vi "Update Params.vi"(6 "EccFileName":string="ocv4.ecc", 7 "Params":T1(array[cluster]), 8 "error in (no error)":errorcluster, 9 "TechIndex":i32, 10 "Channel":u8, 11 "ID":i32) -> (0 "error out":errorcluster, 3 "ID Out":i32)   [LabVIEW 2022 SP3, in "EClib functions.lvlib"]
doc: "This VI stops loaded ecc protocols on the selected channel."
uses:
  EClib functions.lvlib
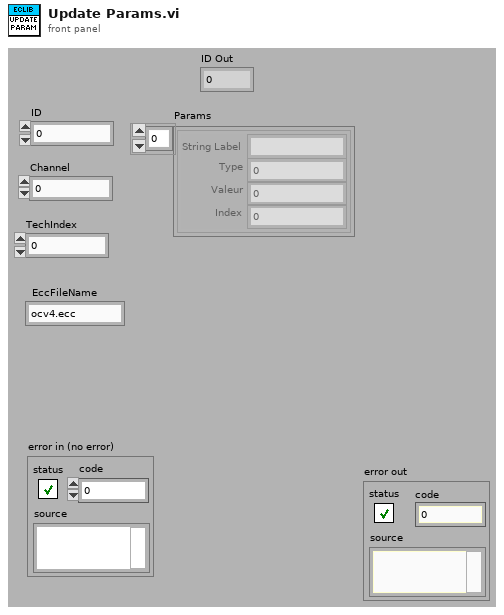
[diagram p1: front panel]
types:
  T1 = cluster{"String Label":string, "Type":i32, "Valeur":i32, "Index":i32}[]
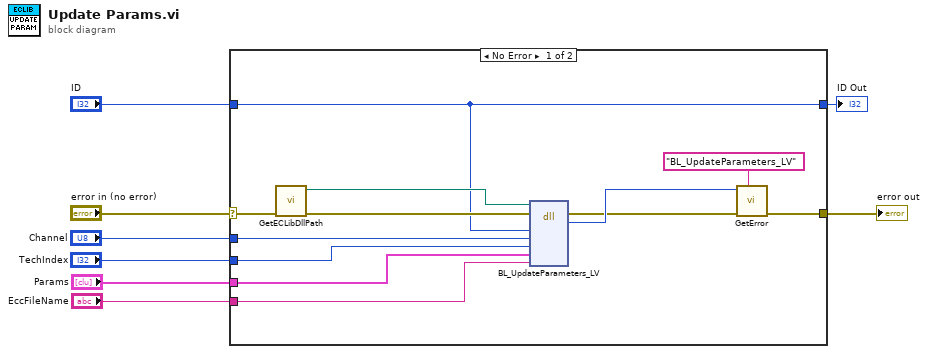
[diagram p0: block diagram]
diagram:
  n1 = case shown="No Error" "error in (no error)" {
    selector: "error in (no error)" -> [w14 w22]
    tunnel: [w19 w22] -> w8
    tunnel: "Params" -> [w13 _]
    tunnel: "TechIndex" -> [w12 _]
    tunnel: "Channel" -> [w11 _]
    tunnel: "EccFileName" -> [w10 _]
    tunnel: "ID" -> [w9 w21]
    tunnel: [w9 w21] -> w1
    frame No Error {
      n2 = call "GetECLibDllPath.vi"("error in (no error)"=w14) -> ("error out"=w15:errorcluster, "ECLibDLLPath"=w20:path)  [unwired: 9 in]
      n3 = dll-call lib="?" fn="BL_UpdateParameters_LV"(path in=w20, error in=w15, "ID"=w9, "Channel"=w11, "TechIndex"=w12, "Params"=w13, "EccFileName"=w10) -> (error out=w16:errorcluster, "return type"=w18:i32)  [unwired: 6 in, 1 out]
      n4 = call "GetError.vi"("DLLFunction"="BL_UpdateParameters_LV", "error in"=w16, "code"=w18) -> ("error out"=w19:errorcluster)  [unwired: 8 in]
    }
    frame Error {
    }
  }
  "error out" <- w8
  "ID Out" <- w1
